vi "Create.vi"(8 "error in (no error)":errorcluster, 10 "Hardware Settings":T1, 11 "Actuator Factory in":refnum<class "Actuator Factory.lvclass">) -> (0 "error out":errorcluster, 2 "Actuator":refnum<class "Actuator.lvclass">, 3 "Actuator Factory out":refnum<class "Actuator Factory.lvclass">)   [LabVIEW 2015, in "Actuator Factory.lvclass"]
uses:
  Actuator Factory.lvclass
  Typedefs/Hardware Settings.ctl
  Typedefs/Actuator Types.ctl
  Typedefs/Cylinder Types.ctl
  Actuator/Actuator.lvclass
  Actuator Cylinder/Actuator Cylinder Factory/Actuator Cylinder Factory.lvclass
  Single Cylinder Actuator/Single Cylinder Actuator.lvclass
  Single Cylinder Actuator/Single Cylinder Actuator.lvclass/Single Cylinder Actuator.ctl
  Dual Cylinder Actuator/Dual Cylinder Actuator.lvclass
  Dual Cylinder Actuator/Dual Cylinder Actuator.lvclass/Dual Cylinder Actuator.ctl
  Dual Cylinder Outer Loop Actuator/Dual Cylinder Outer Loop Actuator.lvclass
  Dual Cylinder Outer Loop Actuator/Dual Cylinder Outer Loop Actuator.lvclass/Dual Cylinder Outer Loop Actuator.ctl
  Boot Loader/Boot Loader.lvclass
  Typedefs/FAMT Typedefs.lvlib
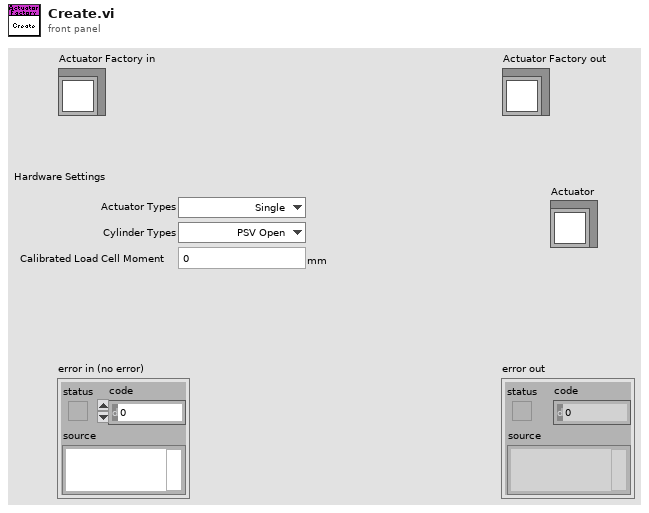
[diagram p1: front panel]
types:
  T1 = typedef "FAMT Typedefs.lvlib/Hardware Settings.ctl" = cluster{"Actuator Types":T2, "Cylinder Types":T3, "Calibrated Load Cell Moment":dbl[unit]}
  T2 = typedef "FAMT Typedefs.lvlib/Actuator Types.ctl" = enum16{"Single", "Dual", "Dual Outer"}
  T3 = typedef "FAMT Typedefs.lvlib/Cylinder Types.ctl" = enum16{"PSV Open", "PSV Closed", "TV Open", "TV Closed", "Closed"}
  T4 = typedef "FAMT Typedefs.lvlib/PID Settings.ctl" = cluster{"Pressure Servo Valve Settings":T5, "Turbo Valve Settings":T5, "Axial Settings":T5, "Lateral Settings":T5}
  T5 = typedef "FAMT Typedefs.lvlib/Closed Loop Settings.ctl" = cluster{"P":dbl, "I":dbl, "D":dbl, "Minimum":dbl, "Maximum":dbl}
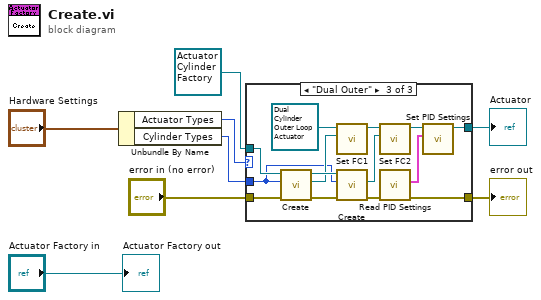
[diagram p0: block diagram]
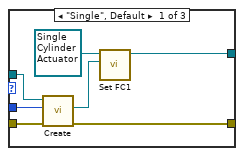
[diagram p2: hidden frame]
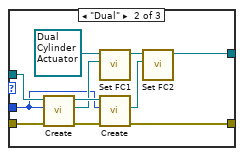
[diagram p3: hidden frame]
diagram:
  n1 = Unbundle By Name("Hardware Settings") -> ("Actuator Types"=w7:T2, "Cylinder Types"=w5:T3)
  n2 = case shown="\"Dual Outer\"" w7 {
    tunnel: refnum<class "Actuator Cylinder Factory.lvclass"> refnum ("ActuatorCylinderFactory.lvclass") -> [w15 w26 w40]
    tunnel: w5 -> [w14 w16 w32]
    tunnel: [w11 w22 w30] -> w4
    tunnel: "error in (no error)" -> [w10 w24 w38]
    tunnel: [w9 w19 w27] -> w1
    frame "Single", Default {
      n3 = call-dynamic "Create.vi"("error in (no error)"=w10, "Cylinder Types"=w14, "Actuator Cylinder Factory in"=w15) -> ("error out"=w11:errorcluster, "Actuator Cylinder"=w13:refnum<class "Actuator Cylinder.lvclass">)  [unwired: 6 in, 1 out]
      n4 = call "Set FC1.vi"("FC1"=w13, "SingleCylinderActuator in"=refnum<class "Single Cylinder Actuator.lvclass"> refnum ("SingleCylinderActuator.lvclass")) -> ("SingleCylinderActuator out"=w9:refnum<class "Single Cylinder Actuator.lvclass">)  [unwired: 9 in]
    }
    frame "Dual" {
      n5 = call-dynamic "Create.vi"("error in (no error)"=w24, "Cylinder Types"=w16, "Actuator Cylinder Factory in"=w26) -> ("error out"=w23:errorcluster, "Actuator Cylinder"=w18:refnum<class "Actuator Cylinder.lvclass">, "Actuator Cylinder Factory out"=w25:refnum<class "Actuator Cylinder Factory.lvclass">)  [unwired: 6 in]
      n6 = call "Set FC1.vi"("FC1"=w18, "SingleCylinderActuator in"=refnum<class "Dual Cylinder Actuator.lvclass"> refnum ("DualCylinderActuator.lvclass")) -> ("SingleCylinderActuator out"=w20:refnum<class "Dual Cylinder Actuator.lvclass">)  [unwired: 9 in]
      n7 = call-dynamic "Create.vi"("error in (no error)"=w23, "Cylinder Types"=w16, "Actuator Cylinder Factory in"=w25) -> ("error out"=w22:errorcluster, "Actuator Cylinder"=w17:refnum<class "Actuator Cylinder.lvclass">)  [unwired: 6 in, 1 out]
      n8 = call "Set FC2.vi"("FC2"=w17, "DualCylinderActuator in"=w20) -> ("DualCylinderActuator out"=w19:refnum<class "Dual Cylinder Actuator.lvclass">)  [unwired: 9 in]
    }
    frame "Dual Outer" {
      n9 = call-dynamic "Create.vi"("error in (no error)"=w38, "Cylinder Types"=w32, "Actuator Cylinder Factory in"=w40) -> ("error out"=w37:errorcluster, "Actuator Cylinder"=w34:refnum<class "Actuator Cylinder.lvclass">, "Actuator Cylinder Factory out"=w39:refnum<class "Actuator Cylinder Factory.lvclass">)  [unwired: 6 in]
      n10 = call "Set FC1.vi"("FC1"=w34, "SingleCylinderActuator in"=refnum<class "Dual Cylinder Outer Loop Actuator.lvclass"> refnum ("DualCylinderActuator.lvclass")) -> ("SingleCylinderActuator out"=w35:refnum<class "Dual Cylinder Outer Loop Actuator.lvclass">)  [unwired: 9 in]
      n11 = call-dynamic "Create.vi"("error in (no error)"=w37, "Cylinder Types"=w32, "Actuator Cylinder Factory in"=w39) -> ("error out"=w31:errorcluster, "Actuator Cylinder"=w33:refnum<class "Actuator Cylinder.lvclass">)  [unwired: 6 in, 1 out]
      n12 = call "Set FC2.vi"("FC2"=w33, "DualCylinderActuator in"=w35) -> ("DualCylinderActuator out"=w28:refnum<class "Dual Cylinder Outer Loop Actuator.lvclass">)  [unwired: 9 in]
      n13 = call "Read PID Settings.vi"("error in (no error)"=w31) -> ("error out"=w30:errorcluster, "PID Settings"=w29:T4)  [unwired: 8 in, 1 out]
      n14 = call "Set PID Settings.vi"("PID Settings"=w29, "Dual Cylinder Outer Loop Actuator in"=w28) -> ("Dual Cylinder Outer Loop Actuator out"=w27:refnum<class "Dual Cylinder Outer Loop Actuator.lvclass">)  [unwired: 9 in]
    }
  }
  "error out" <- w4
  "Actuator" <- w1
  "Actuator Factory out" <- "Actuator Factory in"
